vi "Burst Facade.vi"(0 "Data In":T4={"Active"=FALSE, "Delay (ms)"=0.0, "Duration (ms)"=50.0, "Ramp (ms)"=5.0, "Rate (Hz)"=0.0, "Trepeat (ms)"=0.0, "Repeat"=FALSE}, 2 "Display State In":T2, 3 "Container State":T3) -> (6 "Data Out":T4={"Active"=FALSE, "Delay (ms)"=0.0, "Duration (ms)"=50.0, "Ramp (ms)"=5.0, "Rate (Hz)"=0.0, "Trepeat (ms)"=0.0, "Repeat"=FALSE}, 7 "Display State Out":T2, 8 "Action":T1)   [LabVIEW 2020, in "Burst Control.xctl"]
uses:
  Burst Control.xctl
  Burst Data.ctl
  <vilib>/_xctls/Container State.ctl
  Burst State.ctl
  <vilib>/_xctls/Action.ctl
  <vilib>/_xctls/XControlSupport.lvlib
panel:
  out "conditional display":bool
  in  "Ramp (ms)":dbl
  in  "Duration (ms)":dbl
  in  "Active":bool caption="Gated?"
  in  "Delay (ms)":dbl
  in  "for":dbl caption="ms"
  in  "at":dbl caption="Hz"
  in  "Repeat":bool
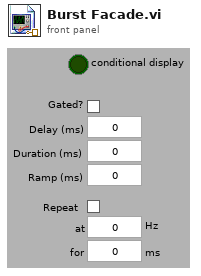
[diagram p1: front panel]
types:
  T1 = typedef "XControlSupport.lvlib/Action.ctl" = cluster{"Data Changed?":bool, "State Changed?":bool, "Action Name":string}
  T2 = typedef "Burst Control.xctl/Burst State.ctl" = cluster{"Numeric":dbl}
  T3 = typedef "XControlSupport.lvlib/Container State.ctl" = cluster{"Indicator?":bool, "Run Mode?":bool, " Refnum":refnum<vi>}
  T4 = typedef "Burst Control.xctl/Burst Data.ctl" = cluster{"Active":bool, "Delay (ms)":dbl, "Duration (ms)":dbl, "Ramp (ms)":dbl, "Rate (Hz)":dbl, "Trepeat (ms)":dbl, "Repeat":bool}
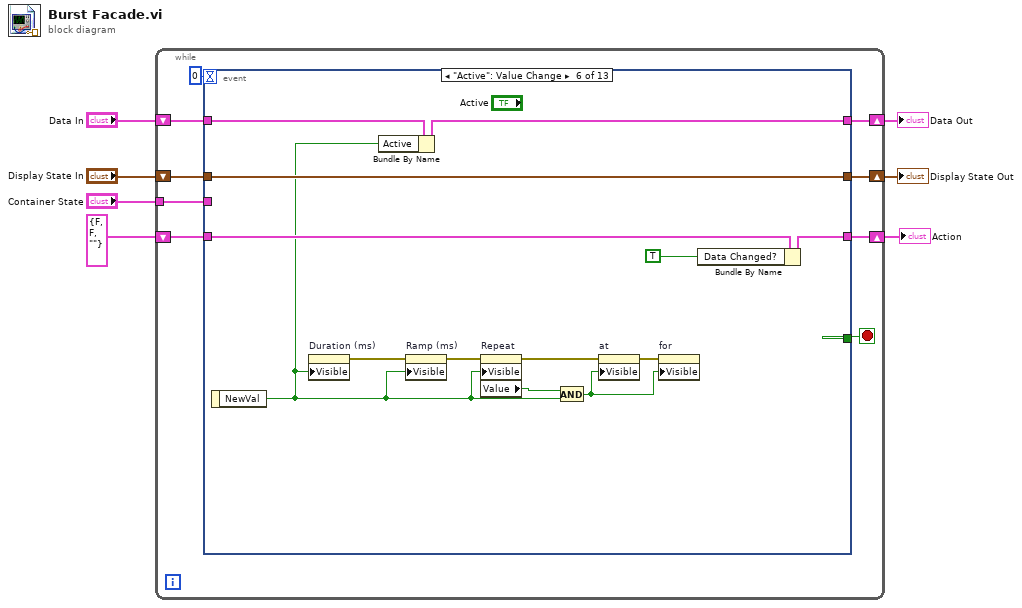
[diagram p0: block diagram]
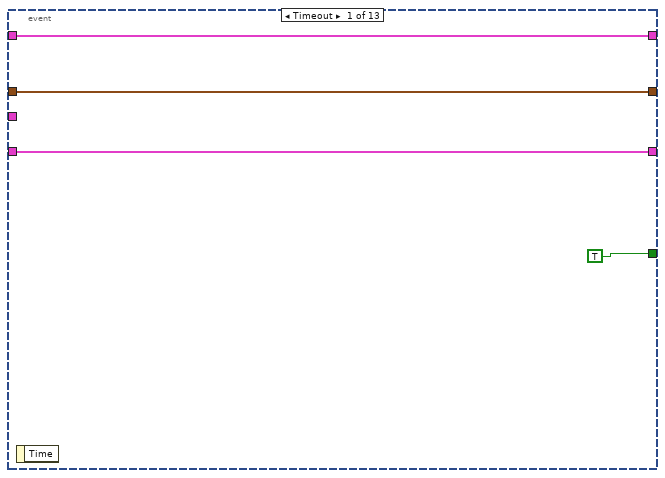
[diagram p2: hidden frame]
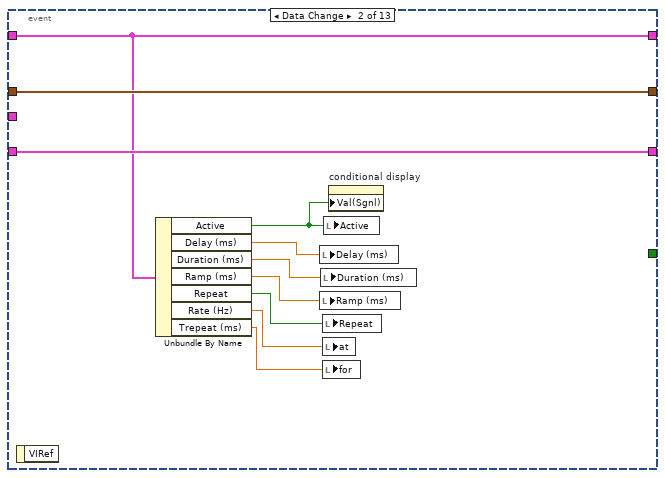
[diagram p3: hidden frame]
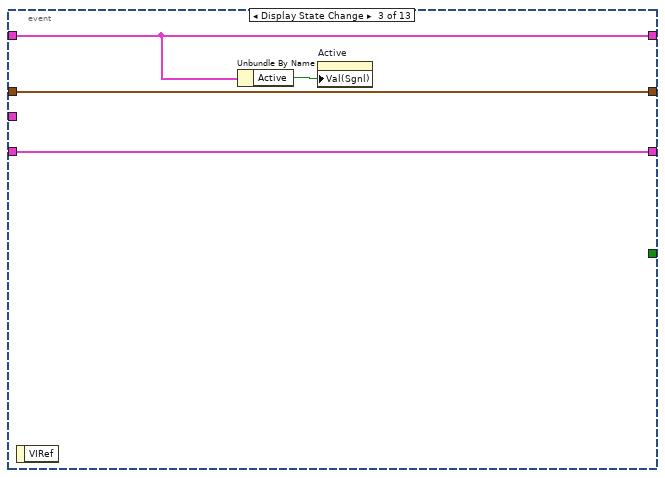
[diagram p4: hidden frame]
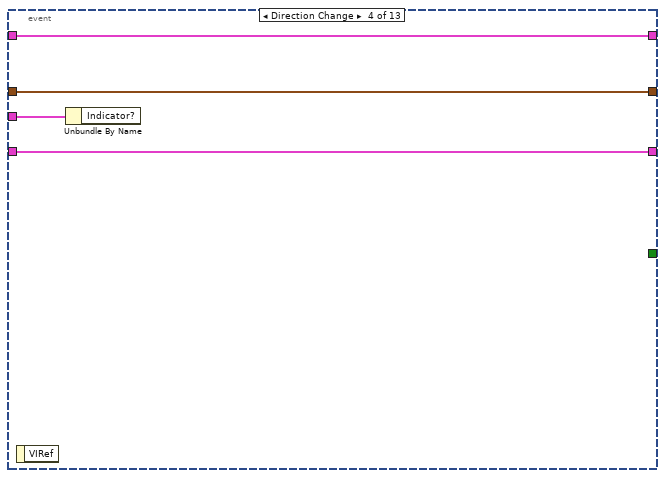
[diagram p5: hidden frame]
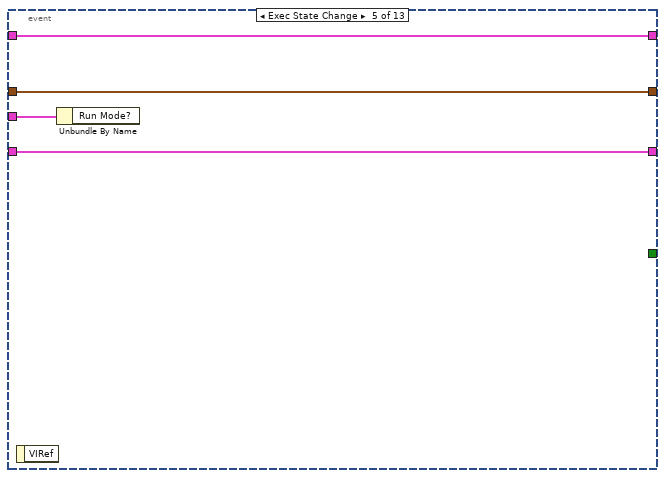
[diagram p6: hidden frame]
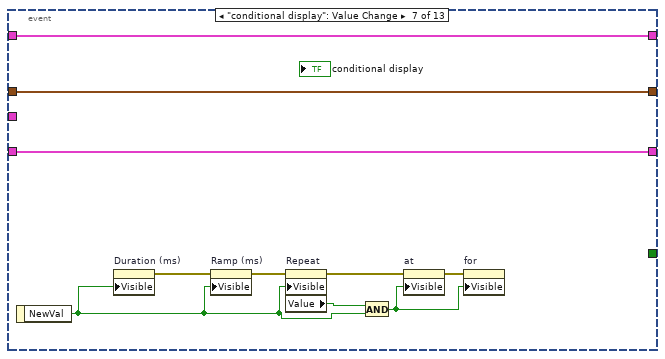
[diagram p7: hidden frame]
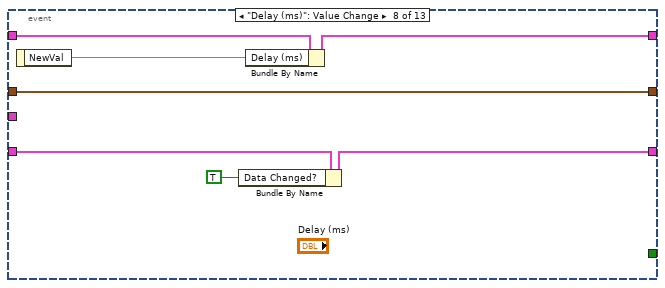
[diagram p8: hidden frame]
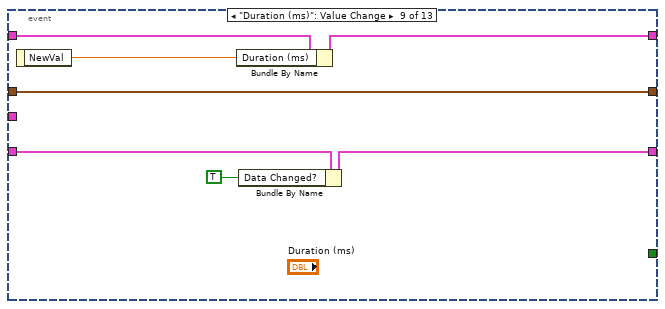
[diagram p9: hidden frame]
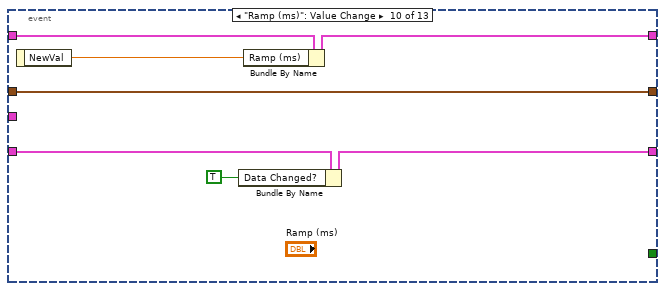
[diagram p10: hidden frame]
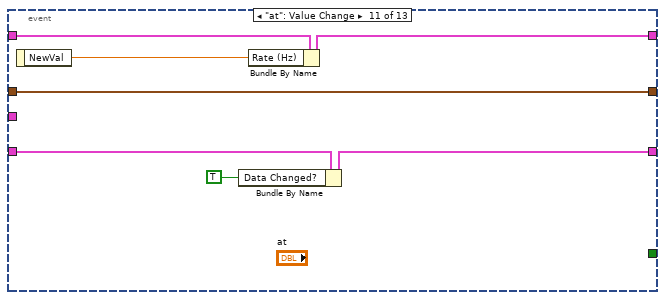
[diagram p11: hidden frame]
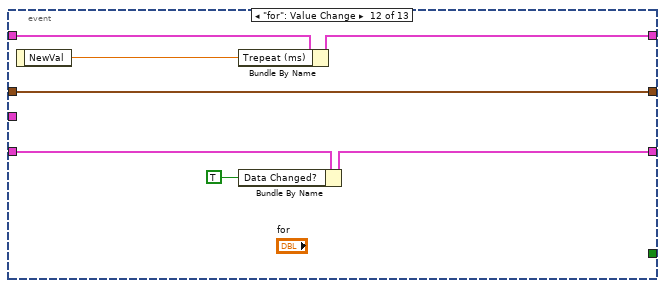
[diagram p12: hidden frame]
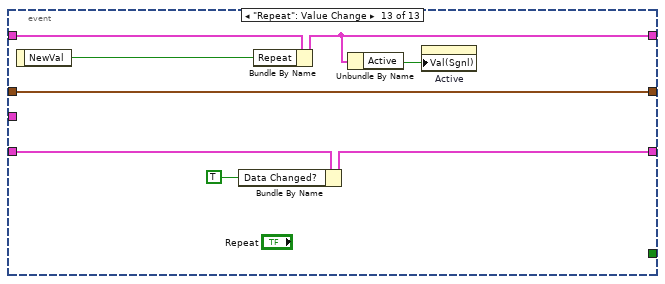
[diagram p13: hidden frame]
diagram:
  n1 = while {
    shift-right: [w15] -> w4
    shift-left: "Display State In" -> [w16]
    tunnel: "Container State" -> [w12]
    shift-right: [w10] -> w7
    shift-left: "Data In" -> [w11]
    shift-right: [w8] -> w2
    shift-left: T1 {"Data Changed?"=FALSE, "State Changed?"=FALSE, "Action Name"=""} ("Action") -> [w9]
    stop <- w14 stop-if-true
    n2 = event shown="[5] \"Active\": Value Change" {
      selector: _ -> [_ _ _ _ _ _ _ _ _ _ _ _ _]
      dyn-events: _ -> [_ _ _ _ _ _ _ _ _ _ _ _ _]
      timeout: 0 -> [_ _ _ _ _ _ _ _ _ _ _ _ _]
      tunnel: w16 -> [w18 w30 w34 w37 w41 w55 w65 w72 w79 w86 w93 w100 w108]
      tunnel: [w18 w30 w34 w37 w41 w55 w65 w72 w79 w86 w93 w100 w108] -> w15
      tunnel: [TRUE _ _ _ _ _ _ _ _ _ _ _ _] -> w14
      tunnel: w12 -> [_ _ _ w38 w42 _ _ _ _ _ _ _ _]
      tunnel: w11 -> [w17 w28 w32 w36 w40 w51 w63 w68 w75 w82 w89 w96 w104]
      tunnel: [w17 w28 w32 w36 w40 w52 w63 w66 w73 w80 w87 w94 w102] -> w10
      tunnel: [w19 w29 w33 w35 w39 w53 w64 w70 w77 w84 w91 w98 w106] -> w8
      tunnel: w9 -> [w19 w29 w33 w35 w39 w54 w64 w71 w78 w85 w92 w99 w107]
      event Timeout {
        n3 = event-data() -> ()  [unwired: 1 in, 1 out]
      }
      event Data Change {
        n4 = event-data() -> ()  [unwired: 1 in, 1 out]
        n5 = Unbundle By Name(w28) -> ("Active"=w21:bool, "Delay (ms)"=w27:dbl, "Duration (ms)"=w26:dbl, "Ramp (ms)"=w25:dbl, "Repeat"=w24:bool, "Rate (Hz)"=w23:dbl, "Trepeat (ms)"=w22:dbl)
        n6 = local write "Delay (ms)"(w27) -> ()
        n7 = local write "Ramp (ms)"(w25) -> ()
        n8 = local write "Duration (ms)"(w26) -> ()
        n9 = local write "Repeat"(w24) -> ()
        n10 = local write "at"(w23) -> ()
        n11 = local write "for"(w22) -> ()
        n12 = local write "Active"(w21) -> ()
        n13 = property on="conditional display" class="Bool (strict)"("Val(Sgnl)"=w21) -> ()  [unwired: 2 in, 2 out]
      }
      event Display State Change {
        n14 = event-data() -> ()  [unwired: 1 in, 1 out]
        n15 = Unbundle By Name(w32) -> ("Active"=w31:bool)
        n16 = property on="Active" class="Bool (strict)"("Val(Sgnl)"=w31) -> ()  [unwired: 2 in, 2 out]
      }
      event Direction Change {
        n17 = event-data() -> ()  [unwired: 1 in, 1 out]
        n18 = Unbundle By Name(w38) -> ()  [unwired: 1 out]
      }
      event Exec State Change {
        n19 = event-data() -> ()  [unwired: 1 in, 1 out]
        n20 = Unbundle By Name(w42) -> ()  [unwired: 1 out]
      }
      event "Active": Value Change {
        n21 = event-data() -> ("NewVal"=w45:bool)  [unwired: 1 in]
        n22 = property on="Duration (ms)" class="DigNum (strict)"("Visible"=w45) -> (error out=w49:errorcluster)  [unwired: 2 in, 1 out]
        n23 = Bundle By Name(cluster=w51, "Active"=w45) -> (w52:T4)
        n24 = property on="Ramp (ms)" class="DigNum (strict)"(error in=w49, "Visible"=w45) -> (error out=w48:errorcluster)  [unwired: 1 in, 1 out]
        n25 = property on="Repeat" class="Bool (strict)"(error in=w48, "Visible"=w45) -> (error out=w47:errorcluster, "Value"=w44:bool)  [unwired: 1 in, 1 out]
        n26 = And(x=w44, y=w45) -> (x .and. y?=w43:bool)
        n27 = property on="at" class="DigNum (strict)"(error in=w47, "Visible"=w43) -> (error out=w46:errorcluster)  [unwired: 1 in, 1 out]
        n28 = property on="for" class="DigNum (strict)"(error in=w46, "Visible"=w43) -> ()  [unwired: 1 in, 2 out]
        n29 = Bundle By Name(cluster=w54, "Data Changed?"=TRUE ("State Changed?")) -> (w53:T1)
      }
      event "conditional display": Value Change {
        n30 = event-data() -> ("NewVal"=w58:bool)  [unwired: 1 in]
        n31 = property on="Duration (ms)" class="DigNum (strict)"("Visible"=w58) -> (error out=w62:errorcluster)  [unwired: 2 in, 1 out]
        n32 = property on="Ramp (ms)" class="DigNum (strict)"(error in=w62, "Visible"=w58) -> (error out=w61:errorcluster)  [unwired: 1 in, 1 out]
        n33 = property on="Repeat" class="Bool (strict)"(error in=w61, "Visible"=w58) -> (error out=w60:errorcluster, "Value"=w56:bool)  [unwired: 1 in, 1 out]
        n34 = And(x=w56, y=w58) -> (x .and. y?=w57:bool)
        n35 = property on="at" class="DigNum (strict)"(error in=w60, "Visible"=w57) -> (error out=w59:errorcluster)  [unwired: 1 in, 1 out]
        n36 = property on="for" class="DigNum (strict)"(error in=w59, "Visible"=w57) -> ()  [unwired: 1 in, 2 out]
      }
      event "Delay (ms)": Value Change {
        n37 = event-data() -> ("NewVal"=w67:dbl)  [unwired: 1 in]
        n38 = Bundle By Name(cluster=w71, "Data Changed?"=TRUE) -> (w70:T1)
        n39 = Bundle By Name(cluster=w68, "Delay (ms)"=w67) -> (w66:T4)
      }
      event "Duration (ms)": Value Change {
        n40 = event-data() -> ("NewVal"=w74:dbl)  [unwired: 1 in]
        n41 = Bundle By Name(cluster=w75, "Duration (ms)"=w74) -> (w73:T4)
        n42 = Bundle By Name(cluster=w78, "Data Changed?"=TRUE) -> (w77:T1)
      }
      event "Ramp (ms)": Value Change {
        n43 = event-data() -> ("NewVal"=w81:dbl)  [unwired: 1 in]
        n44 = Bundle By Name(cluster=w85, "Data Changed?"=TRUE) -> (w84:T1)
        n45 = Bundle By Name(cluster=w82, "Ramp (ms)"=w81) -> (w80:T4)
      }
      event "at": Value Change {
        n46 = event-data() -> ("NewVal"=w88:dbl)  [unwired: 1 in]
        n47 = Bundle By Name(cluster=w92, "Data Changed?"=TRUE) -> (w91:T1)
        n48 = Bundle By Name(cluster=w89, "Rate (Hz)"=w88) -> (w87:T4)
      }
      event "for": Value Change {
        n49 = event-data() -> ("NewVal"=w95:dbl)  [unwired: 1 in]
        n50 = Bundle By Name(cluster=w96, "Trepeat (ms)"=w95) -> (w94:T4)
        n51 = Bundle By Name(cluster=w99, "Data Changed?"=TRUE) -> (w98:T1)
      }
      event "Repeat": Value Change {
        n52 = event-data() -> ("NewVal"=w103:bool)  [unwired: 1 in]
        n53 = Bundle By Name(cluster=w107, "Data Changed?"=TRUE) -> (w106:T1)
        n54 = Bundle By Name(cluster=w104, "Repeat"=w103) -> (w102:T4)
        n55 = Unbundle By Name(w102) -> ("Active"=w101:bool)
        n56 = property on="Active" class="Bool (strict)"("Val(Sgnl)"=w101) -> ()  [unwired: 2 in, 2 out]
      }
    }
  }
  "Display State Out" <- w4
  "Data Out" <- w7
  "Action" <- w2
